vi "RobotMap.vi"() -> ()   [LabVIEW 2018]
uses:
  <vilib>/Rock Robotics/SystemInterfaces/AI/FPGA_AIGyroChannel.ctl
panel:
  in  "Gyro":T1
  in  "4Bar Limit Switch BottomDIO":dbl
  in  "RightDriveSlave2":u8=10
  in  "LeftDriveSlave2":u8=3
  in  "Cargo Intake":dbl=5.0
  in  "Hatch Panel Intake":dbl=6.0
  in  "4BarSlave":u8=7
  in  "4BarMaster":u8=4
  in  "RightDriveSlave1":u8=9
  in  "RightDriveMaster":u8=8
  in  "LeftDriveSlave1":u8=2
  in  "LeftDriveMaster":u8=1
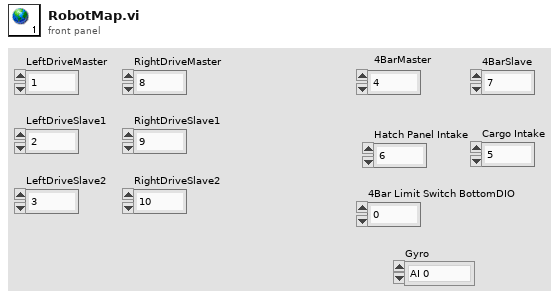
[diagram p1: front panel]
types:
  T1 = typedef "FPGA_AIGyroChannel.ctl" = enum8{"AI 0", "AI 1", "Invalid"}
diagram:
